vi "fg_listbox_sizes.vi"(8 "error in (no error)":errorcluster, 10 "scrollbar_size in":u32=2, 11 "line_size in":u32=2) -> (0 "error out":errorcluster, 2 "scrollbar_size out":u32=2, 3 "line_size out":u32=2)   [LabVIEW 2015, in "lv-pagination.lvlib"]
doc: "This functional global provides a way to configure \"padding\" for calculating the visible cells, you can configure the line size (between cells) and the scrollbar size."
uses:
  lv-pagination.lvlib
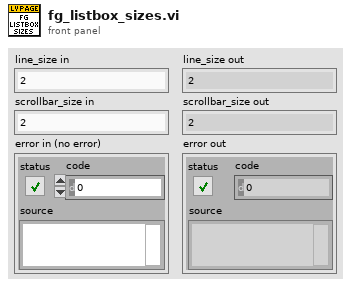
[diagram p1: front panel]
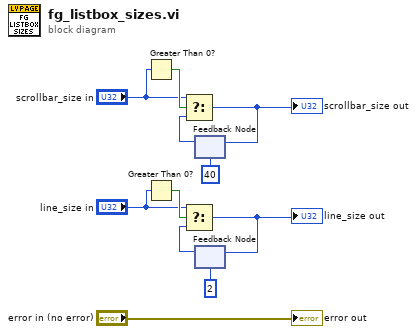
[diagram p0: block diagram]
diagram:
  n1 = Greater Than 0?(x="scrollbar_size in") -> (x > 0?=w6:bool)
  n2 = Greater Than 0?(x="line_size in") -> (x > 0?=w11:bool)
  n3 = feedback #1(u32 40 ("x")) -> (w4:u32)
  n4 = Select(t="scrollbar_size in", s=w6, f=w4) -> (s? t:f=w2:u32)
  "scrollbar_size out" <- w2
  n5 = feedback-in #1(w2) -> ()
  n6 = feedback #2(u32 2 ("x")) -> (w8:u32)
  n7 = Select(t="line_size in", s=w11, f=w8) -> (s? t:f=w9:u32)
  "line_size out" <- w9
  n8 = feedback-in #2(w9) -> ()
  "error out" <- "error in (no error)"
